vi "GetM100PassFailYield.vi"(10 "RCNO":string="A150100736") -> (0 "Step":string, 1 "Yield":dbl, 2 "Fail":i32, 3 "Pass":i32, 4 "待測":i32, 6 "已測":i32)   [LabVIEW 2012]
uses:
  <vilib>/addons/database/Auxilliary.llb/DB Tools Cursor Type.ctl
  <vilib>/addons/database/Connection.llb/DB Tools Open Connec (Path).vi
  <vilib>/addons/database/Connection.llb/Conn Execute.vi
  <vilib>/addons/database/Recordset.llb/Rec Fetch Integer Data (R).vi
  <vilib>/addons/database/Recordset.llb/Rec Destroy - Connection.vi
  <vilib>/addons/database/Recordset.llb/Rec Fetch String Data (R).vi
  <vilib>/addons/database/NI_Database_API.lvlib
panel:
  out "ReceiveQty":i32
  out "concatenated string 2":string
  out "concatenated string":string
  out "error out":errorcluster
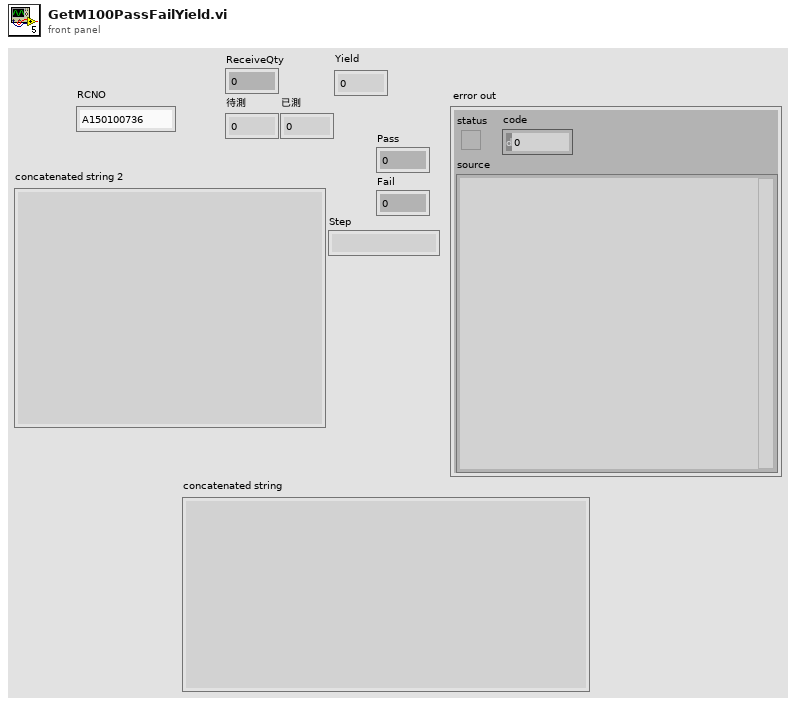
[diagram p1: front panel]
types:
  T1 = typedef "NI_Database_API.lvlib/DB Tools Cursor Type.ctl" = enum16{"forward-only", "keyset", "dynamic", "static"}
  T2 = typedef "NI_Database_API.lvlib/Conn ObjectReference.ctl" = refnum<k1>
  T3 = typedef "NI_Database_API.lvlib/Rec ObjectReference.ctl" = refnum<k1>
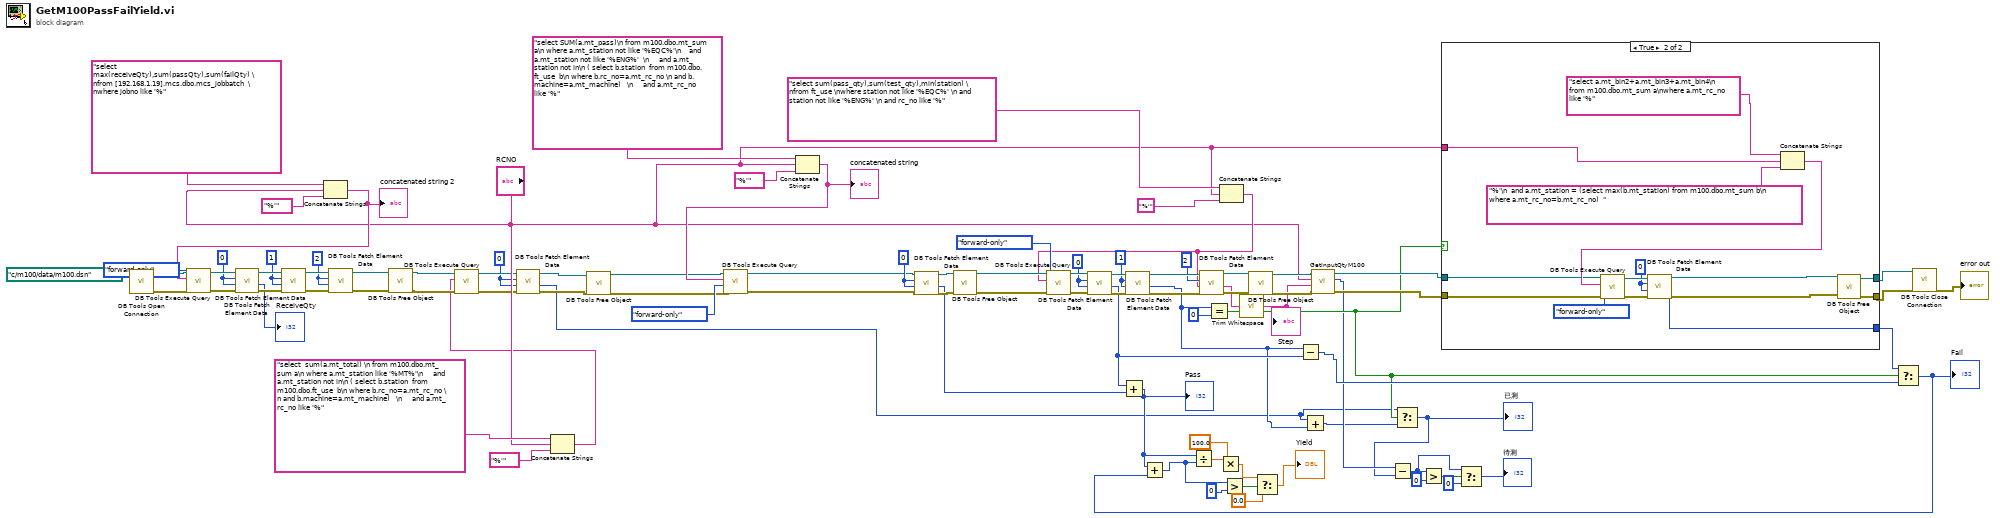
[diagram p0: block diagram]
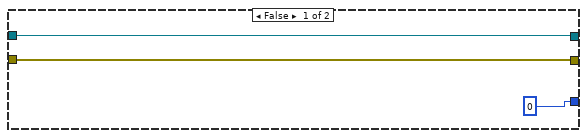
[diagram p2: hidden frame]
diagram:
  w18 = 0
  w57 = 2
  w58 = 1
  w59 = 0
  w72 = 1
  w73 = 0
  w90 = 0
  n1 = call-poly <vilib>:"DB Tools Open Connection.vi"("connection information"=path "c:/m100/data/m100.dsn") -> ("error out"=w67:errorcluster, "connection reference"=w68:T2)  [unwired: 7 in]
  n2 = Concatenate Strings("select max(receiveQty),sum(passQty),sum(failQty) \nfrom [192.168.1.19].mcs.dbo.mcs_jobbatch  \nwhere jobno like '%", "RCNO", "%'" ("string")) -> (w69:string)
  "concatenated string 2" <- w69
  n3 = call-poly <vilib>:"DB Tools Execute Query.vi"("error in (no error)"=w67, "cursor type"=DB_Tools_Cursor_Type."forward-only", "SQL query"=w69, "connection reference"=w68) -> ("error out"=w64:errorcluster, "recordset reference"=w65:T3)  [unwired: 4 in]
  n4 = call-poly <vilib>:"DB Tools Fetch Element Data.vi"("error in (no error)"=w64, "type"=w59, "column index"=w59, "recordset reference"=w65) -> ("error out"=w63:errorcluster, "data"=→"ReceiveQty":i32, "recordset reference out"=w62:T3)  [unwired: 3 in]
  n5 = call-poly <vilib>:"DB Tools Fetch Element Data.vi"("error in (no error)"=w63, "type"=w58, "column index"=w58, "recordset reference"=w62) -> ("error out"=w61:errorcluster, "recordset reference out"=w60:T3)  [unwired: 3 in, 1 out]
  n6 = call-poly <vilib>:"DB Tools Fetch Element Data.vi"("error in (no error)"=w61, "type"=w57, "column index"=w57, "recordset reference"=w60) -> ("error out"=w55:errorcluster, "recordset reference out"=w56:T3)  [unwired: 3 in, 1 out]
  n7 = call-poly <vilib>:"DB Tools Free Object.vi"("error in (no error)"=w55, "recordset reference"=w56) -> ("error out"=w28:errorcluster, "connection reference"=w29:T2)  [unwired: 8 in]
  n8 = Concatenate Strings("select  sum(a.mt_total) \n from m100.dbo.mt_sum a\n where a.mt_station like '%MT%'\n     and a.mt_station not in\n ( select b.station  from m100.dbo.ft_use  b\n where b.rc_no=a.mt_rc_no \n and b.machine=a.mt_machine)   \n     and a.mt_rc_no like '%", "RCNO", "%'" ("string")) -> (w17:string)
  n9 = call-poly <vilib>:"DB Tools Execute Query.vi"("error in (no error)"=w28, "SQL query"=w17, "connection reference"=w29) -> ("error out"=w23:errorcluster, "recordset reference"=w24:T3)  [unwired: 5 in]
  n10 = call-poly <vilib>:"DB Tools Fetch Element Data.vi"("error in (no error)"=w23, "type"=w18, "column index"=w18, "recordset reference"=w24) -> ("error out"=w21:errorcluster, "data"=w1:i32, "recordset reference out"=w22:T3)  [unwired: 3 in]
  n11 = call-poly <vilib>:"DB Tools Free Object.vi"("error in (no error)"=w21, "recordset reference"=w22) -> ("error out"=w19:errorcluster, "connection reference"=w20:T2)  [unwired: 8 in]
  n12 = Concatenate Strings("select SUM(a.mt_pass)\n from m100.dbo.mt_sum a\n where a.mt_station not like '%EQC%'\n    and a.mt_station not like '%ENG%'  \n     and a.mt_station not in\n ( select b.station  from m100.dbo.ft_use  b\n where b.rc_no=a.mt_rc_no \n and b.machine=a.mt_machine)   \n     and a.mt_rc_no like '%", "RCNO", "%'" ("string")) -> (w85:string)
  "concatenated string" <- w85
  n13 = call-poly <vilib>:"DB Tools Execute Query.vi"("error in (no error)"=w19, "cursor type"=DB_Tools_Cursor_Type."forward-only", "SQL query"=w85, "connection reference"=w20) -> ("error out"=w15:errorcluster, "recordset reference"=w16:T3)  [unwired: 4 in]
  n14 = call-poly <vilib>:"DB Tools Fetch Element Data.vi"("error in (no error)"=w15, "type"=w90, "column index"=w90, "recordset reference"=w16) -> ("error out"=w88:errorcluster, "data"=w41:i32, "recordset reference out"=w89:T3)  [unwired: 3 in]
  n15 = call-poly <vilib>:"DB Tools Free Object.vi"("error in (no error)"=w88, "recordset reference"=w89) -> ("error out"=w80:errorcluster, "connection reference"=w82:T2)  [unwired: 8 in]
  n16 = Concatenate Strings("select sum(pass_qty),sum(test_qty),min(station) \nfrom ft_use \nwhere station not like '%EQC%' \n and station not like '%ENG%' \n and rc_no like '%" ("SQL query"), "RCNO", "%'" ("string")) -> (w49:string)
  n17 = call-poly <vilib>:"DB Tools Execute Query.vi"("error in (no error)"=w80, "cursor type"=DB_Tools_Cursor_Type."forward-only", "SQL query"=w49, "connection reference"=w82) -> ("error out"=w79:errorcluster, "recordset reference"=w81:T3)  [unwired: 4 in]
  n18 = call-poly <vilib>:"DB Tools Fetch Element Data.vi"("error in (no error)"=w79, "type"=w73, "column index"=w73, "recordset reference"=w81) -> ("error out"=w75:errorcluster, "data"=w39:i32, "recordset reference out"=w74:T3)  [unwired: 3 in]
  n19 = Add(x=w39, y=w41) -> (x+y=w13:i32)
  "Pass" <- w13
  n20 = call-poly <vilib>:"DB Tools Fetch Element Data.vi"("error in (no error)"=w75, "type"=w72, "column index"=w72, "recordset reference"=w74) -> ("error out"=w52:errorcluster, "data"=w2:i32, "recordset reference out"=w54:T3)  [unwired: 3 in]
  n21 = call-poly <vilib>:"DB Tools Fetch Element Data.vi"("error in (no error)"=w52, "type"=w49, "column index"=2, "recordset reference"=w54) -> ("error out"=w51:errorcluster, "data"=w44:string, "recordset reference out"=w53:T3)  [unwired: 3 in]
  n22 = Equal?(x=w2, y=0) -> (x = y?=w36:bool)
  n23 = call <vilib>:"Trim Whitespace.vi"("string"=w44) -> ("trimmed string"=w43:string)  [unwired: 1 in]
  "Step" <- w43
  n24 = call-poly <vilib>:"DB Tools Free Object.vi"("error in (no error)"=w51, "recordset reference"=w53) -> ("error out"=w47:errorcluster, "connection reference"=w48:T2)  [unwired: 8 in]
  n25 = Subtract(x=w2, y=w39) -> (x-y=w37:i32)
  n26 = Add(x=w1, y=w2) -> (x+y=w3:i32)
  n27 = call "GetInputQtyM100.vi"("error in (no error)"=w47, "Step"=w43, "RCNO"="RCNO", "connection reference"=w48) -> ("error out"=w45:errorcluster, "InputQty"=w35:i32, "connection reference 2"=w46:T2)  [unwired: 5 in]
  n28 = Select(t=w1, s=w36, f=w3) -> (s? t:f=w10:i32)
  "已測" <- w10
  n29 = Subtract(x=w35, y=w10) -> (x-y=w32:i32)
  n30 = Greater?(x=w32, y=0) -> (0:w33:bool)
  n31 = case shown="True" w36 {
    tunnel: [w96 w108] -> w87
    tunnel: [w95 w107] -> w86
    tunnel: "RCNO" -> [_ w102]
    tunnel: w46 -> [w96 w101]
    tunnel: w45 -> [w95 w100]
    tunnel: [0 ("data") w97] -> w38
    frame False {
    }
    frame True {
      w109 = 0
      n32 = Concatenate Strings("select a.mt_bin2+a.mt_bin3+a.mt_bin4\n   from m100.dbo.mt_sum a\nwhere a.mt_rc_no like '%" ("SQL query"), w102, "%'\n  and a.mt_station = (select max(b.mt_station) from m100.dbo.mt_sum b\n                      where a.mt_rc_no=b.mt_rc_no)  " ("SQL query")) -> (w103:string)
      n33 = call-poly <vilib>:"DB Tools Execute Query.vi"("error in (no error)"=w100, "cursor type"=DB_Tools_Cursor_Type."forward-only", "SQL query"=w103, "connection reference"=w101) -> ("error out"=w110:errorcluster, "recordset reference"=w111:T3)  [unwired: 4 in]
      n34 = call-poly <vilib>:"DB Tools Fetch Element Data.vi"("error in (no error)"=w110, "type"=w109, "column index"=w109, "recordset reference"=w111) -> ("error out"=w98:errorcluster, "data"=w97:i32, "recordset reference out"=w99:T3)  [unwired: 3 in]
      n35 = call-poly <vilib>:"DB Tools Free Object.vi"("error in (no error)"=w98, "recordset reference"=w99) -> ("error out"=w107:errorcluster, "connection reference"=w108:T2)  [unwired: 8 in]
    }
  }
  n36 = Select(t=w32, s=w33, f=0) -> (s? t:f=→"待測":i32)
  n37 = Select(t=w38, s=w36, f=w37) -> (s? t:f=w14:i32)
  "Fail" <- w14
  n38 = Add(x=w13, y=w14) -> (x+y=w9:i32)
  n39 = Divide(x=w13, y=w9) -> (x/y=w12:dbl)
  n40 = Multiply(x=w12, y=100.0) -> (x*y=w6:dbl)
  n41 = Greater?(x=w9, y=0) -> (0:w7:bool)
  n42 = Select(t=w6, s=w7, f=0.0) -> (s? t:f=→"Yield":dbl)
  n43 = call <vilib>:"DB Tools Close Connection.vi"("error in (no error)"=w86, "connection reference"=w87) -> ("error out"=→"error out":errorcluster)  [unwired: 5 in]
